vi "array to general.vi"(1 "TP Information out":string[](array[string])) -> (0 "字符串":string)   [LabVIEW 2018]
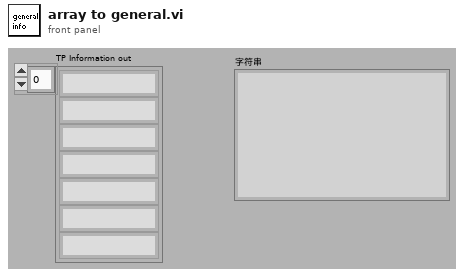
[diagram p1: front panel]
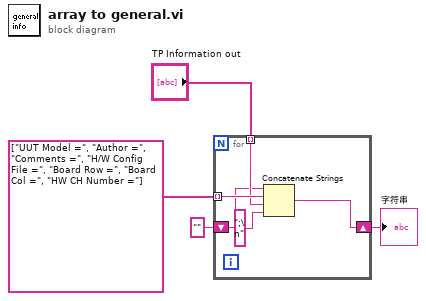
[diagram p0: block diagram]
diagram:
  n1 = for {
    tunnel: string[] ["UUT Model =", "Author =", "Comments =", "H/W Config File =", "Board Row =", "Board Col =", "HW CH Number ="] -> [w9] mode=indexing
    shift-right: [w6] -> w4
    shift-left: "" -> [w5]
    tunnel: "TP Information out" -> [w8] mode=indexing
    n2 = Concatenate Strings(w5, w9, w8, ";\n" ("元素")) -> (w6:string)
  }
  "字符串" <- w4
